vi "load and intialize target with engines (config out).vi"(6 "timeout in ms (-1)":i32=-1, 8 "error in":errorcluster, 9 "engine aliases (empty = ALL)":string[](array[string]), 10 "target alias":string, 11 "file path":path) -> (0 "error out":errorcluster, 2 "engine runtime interfaces":refnum<class "Engine Runtime Interface.lvclass">[](array[class]), 3 "target runtime":refnum<class "PL_Target Runtime.lvclass">, 4 "filtered engines":T1[](array[typedef]))   [LabVIEW 2015, in "Sequencer Module tests.lvlib"]
doc: "Loads and initializes the target specified by 'target alias' for the configuration file specified by 'file path'. This VI returns an initialized target object with an array of engine objects which can be interacted with using the Engine Execution Interface APIs."
uses:
  Sequencer Module tests.lvlib
  <vilib>/NI/DCAF/Tag Editor Core/Framework Configuration Classes/target runtime/PL_Target Runtime.lvclass
  <vilib>/NI/Module Execution Interface/Engine Runtime/Engine Runtime Interface.lvclass
  <vilib>/NI/DCAF/Tag Editor Core/Framework Configuration Classes/platypus configuration/engines cluster.ctl
  <vilib>/NI/Module Execution Interface/Engine Configuration/engine configuration.lvclass
  <vilib>/NI/Tag Bus Module Framework/module configuration/TBM module configuration.lvclass
  <vilib>/NI/DCAF/Tag Editor Core/Framework Configuration Classes/platypus configuration/PLConfigurationSerializer.lvlib
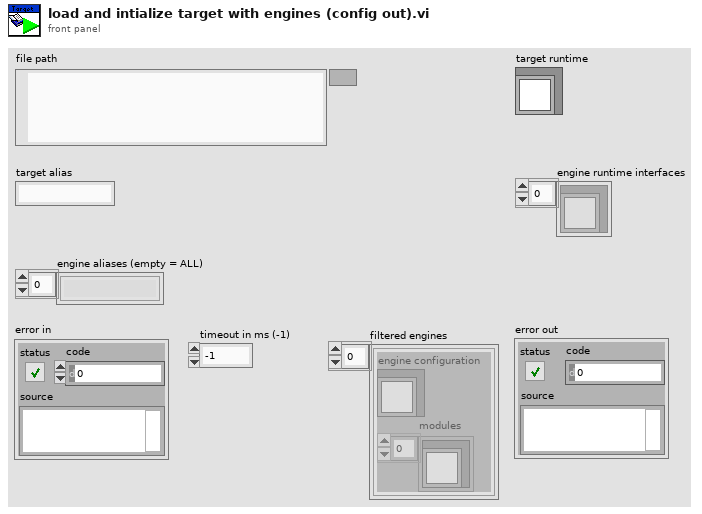
[diagram p1: front panel]
types:
  T1 = typedef "PLConfigurationSerializer.lvlib/engines cluster.ctl" = cluster{"engine configuration":refnum<class "engine configuration.lvclass">, "modules":refnum<class "TBM module configuration.lvclass">[]}
  T2 = typedef "PLConfigurationSerializer.lvlib/targets cluster.ctl" = cluster{"Target Configuration":refnum<class "PL_Target Configuration.lvclass">, "engines":T1[]}
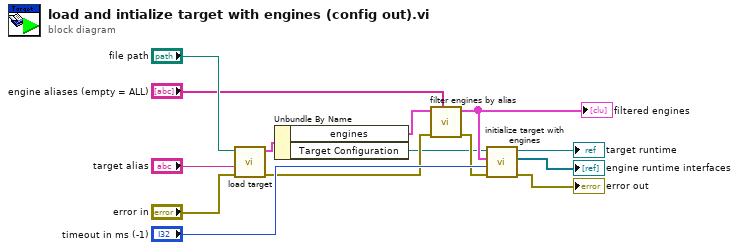
[diagram p0: block diagram]
diagram:
  n1 = call <vilib>:"load target.vi"("error in (no error)"="error in", "target alias"="target alias", "file path"="file path") -> ("error out"=w4:errorcluster, "targets cluster out"=w6:T2)  [unwired: 7 in]
  n2 = Unbundle By Name(w6) -> ("engines"=w5:T1[], "Target Configuration"=w1:refnum<class "PL_Target Configuration.lvclass">)
  n3 = call <vilib>:"filter engines by alias.vi"("engine aliases (empty = ALL)"="engine aliases (empty = ALL)", "error in (no error)"=w4, "target engines"=w5) -> ("error out"=w3:errorcluster, "filtered engines"=w2:T1[])  [unwired: 7 in]
  "filtered engines" <- w2
  n4 = call <vilib>:"initialize target with engines.vi"("error in (no error)"=w3, "timeout in ms (-1)"="timeout in ms (-1)", "engines"=w2, "PL_Target Configuration in"=w1) -> ("error out"=→"error out":errorcluster, "engine runtime interfaces"=→"engine runtime interfaces":refnum<class "Engine Runtime Interface.lvclass">[], "target runtime"=→"target runtime":refnum<class "PL_Target Runtime.lvclass">)  [unwired: 5 in]
